vi "StatMon_StartWarning.vi"() -> (0 "String":string)   [LabVIEW 2016]
uses:
  Instrument_Setup.vi
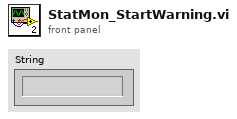
[diagram p1: front panel]
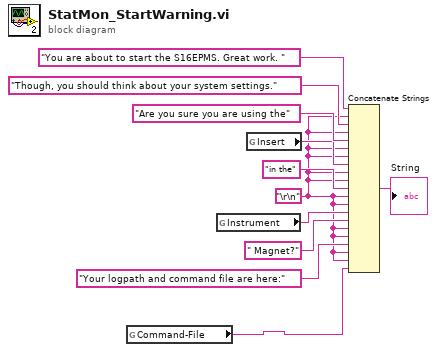
[diagram p0: block diagram]
diagram:
  w2 = "\r\n"
  n1 = global read "Instrument_Setup.vi" "Command-File"() -> (w1:string)
  n2 = global read "Instrument_Setup.vi" "Instrument"() -> (w6:string)
  n3 = global read "Instrument_Setup.vi" "Insert"() -> (w8:string)
  n4 = Concatenate Strings("You are about to start the S16EPMS. Great work. ", w2, "Though, you should think about your system settings.", w2, "Are you sure you are using the", w2, w2, w8, w2, w2, "in the", w2, w2, w6, " Magnet?", w2, w2, "Your logpath and command file are here:", w2, w2, w1) -> (→"String":string)
